vi "Phasor Measurement.vi"(0 "data in":T3, 1 "frequency configuration":T1={"channel index"=0, "nominal Fs/actual Fs"=1.0}, 2 "reset? (F)":bool, 7 "max time error [s]":dbl=1e-07 format="%#_15f", 9 "system info in":refnum<class "PMU System Info.lvclass">, 11 "error in (no error)":errorcluster, 12 "GPS information":T5[](array[typedef])) -> (3 "samples to read":u32, 4 "reporting data":T2 {"frequency" format="%#.6g"}, 6 "reporting timing information":T4 {"time quality flag" format="%.0b"}, 10 "system info out":refnum<class "PMU System Info.lvclass">, 14 "physical phasors":csg[](array[numeric]), 15 "error out":errorcluster)   [LabVIEW 2013, in "NI_EP_PMU.lvlib"]
doc: "LabVIEW no longer supports this VI. Use the Phasor Measurement (Std 2011) VI instead.\n\nCalculates the phasors, frequency, and frequency rate-of-change at the reporting timestamp according to IEEE Std C37.118-2005. This VI also returns the reported timestamp and other timing information for the fields in data frame, configuration frame, header frame, and command frame, as defined in IEEE Std C37.118-2005."
uses:
  <vilib>/addons/Electrical Power/PMU/NI_EP_PMU.lvlib
  <vilib>/addons/Electrical Power/PMU/Common/Classes/PMU System Info/PMU System Info.lvclass
  <vilib>/addons/Electrical Power/PMU/Common/Controls/pmu_GPS Info.ctl
  <vilib>/addons/Electrical Power/PMU/Common/Controls/pmu_Reporting Time Information.ctl
  <vilib>/addons/Electrical Power/PMU/Common/Controls/pmu_Phasor Measurement Data.ctl
  <vilib>/addons/Electrical Power/PMU/Common/Controls/pmu_Reporting Data.ctl
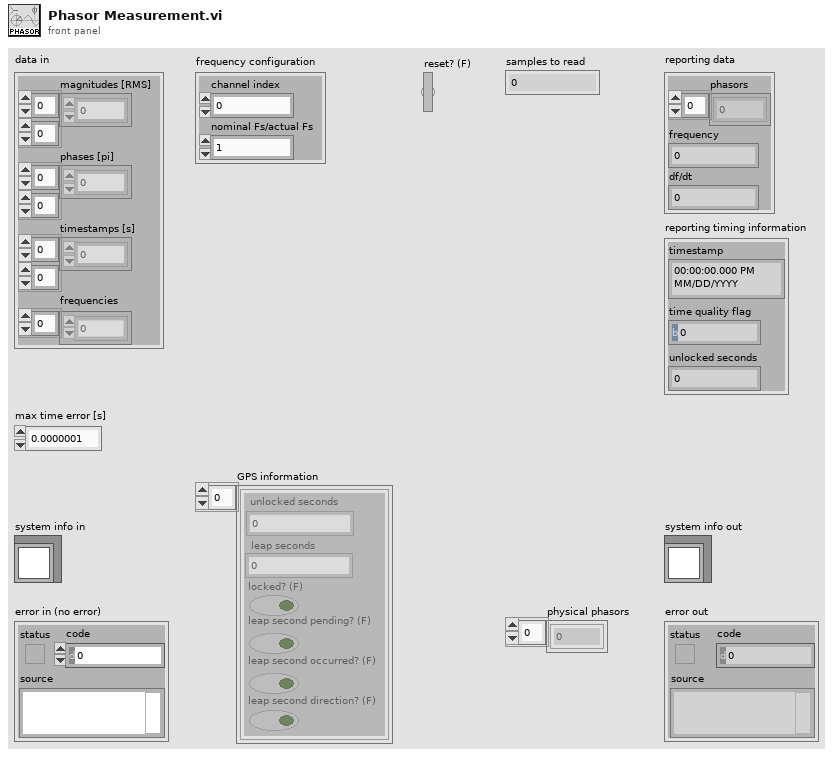
[diagram p1: front panel]
types:
  T1 = cluster{"channel index":i32, "nominal Fs/actual Fs":dbl}
  T2 = typedef "NI_EP_PMU.lvlib/pmu_Reporting Data.ctl" = cluster{"phasors":csg[], "frequency":sgl, "df/dt":sgl}
  T3 = typedef "NI_EP_PMU.lvlib/pmu_Phasor Measurement Data.ctl" = cluster{"magnitudes [RMS]":dbl[][], "phases [pi]":dbl[][], "timestamps [s]":dbl[][], "frequencies":dbl[]}
  T4 = typedef "NI_EP_PMU.lvlib/pmu_Reporting Time Information.ctl" = cluster{"time quality flag":u8, "unlocked seconds":u32, "timestamp":timestamp}
  T5 = typedef "NI_EP_PMU.lvlib/pmu_GPS Info.ctl" = cluster{"unlocked seconds":u32, "leap seconds":i8, "locked? (F)":bool, "leap second pending? (F)":bool, "leap second occurred? (F)":bool, "leap second direction? (F)":bool}
  T6 = cluster{"reporting timestamp":dbl[], "reporting magnitudes [RMS]":dbl[], "reporting phases [pi]":dbl[]}
  T7 = cluster{"zero-crossing timestamps [s]":dbl[], "zero-crossing frequencies":dbl[]}
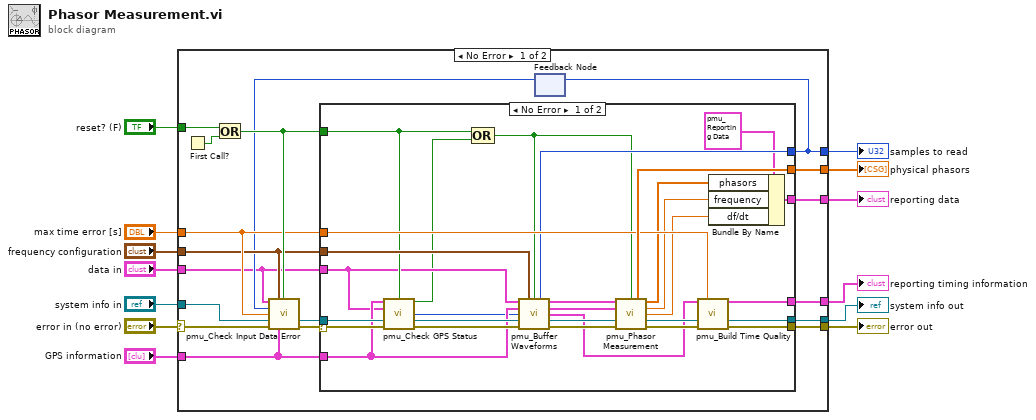
[diagram p0: block diagram]
diagram:
  n1 = case shown="No Error" "error in (no error)" {
    selector: "error in (no error)" -> [w18 w64]
    tunnel: "data in" -> [w14 _]
    tunnel: "system info in" -> [w23 w63]
    tunnel: [w31 _] -> w11
    tunnel: [w30 w63] -> w2
    tunnel: [w29 w64] -> w10
    tunnel: [w28 _] -> w9
    tunnel: "max time error [s]" -> [w24 _]
    tunnel: "frequency configuration" -> [w20 _]
    tunnel: [w16 _] -> w6
    tunnel: "GPS information" -> [w21 _]
    tunnel: "reset? (F)" -> [w26 _]
    tunnel: [w15 _] -> w1
    frame No Error {
      n2 = First Call?() -> (First Call?: T/F=w27:bool)
      n3 = Or(x=w26, y=w27) -> (x .or. y?=w25:bool)
      n4 = feedback #1() -> (w17:u32)  [unwired: 1 in]
      n5 = call <vilib>:"pmu_Check Input Data Error.vi"("data in"=w14, "frequency configuration"=w20, "reset? (F)"=w25, "elements need to read"=w17, "max time error [s]"=w24, "system info in"=w23, "error in (no error)"=w18, "GPS information"=w21) -> ("system info out"=w22:refnum<class "PMU System Info.lvclass">, "error out"=w19:errorcluster)  [unwired: 6 in]
      n6 = case shown="No Error" w19 {
        selector: w19 -> [w44 w62]
        tunnel: w14 -> [w33 _]
        tunnel: [w58 _] -> w31
        tunnel: [w57 w61] -> w30
        tunnel: [w56 w62] -> w29
        tunnel: [w55 _] -> w28
        tunnel: w24 -> [w52 _]
        tunnel: w20 -> [w50 _]
        tunnel: [w42 _] -> w16
        tunnel: w21 -> [w43 _]
        tunnel: w25 -> [w36 _]
        tunnel: w22 -> [w46 w61]
        tunnel: [w37 _] -> w15
        frame No Error {
          n7 = call <vilib>:"pmu_Check GPS Status.vi"("GPS information"=w43, "reset? (F)"=w36, "data in"=w33, "system info in"=w46, "error in (no error)"=w44) -> ("GPS first locking?"=w32:bool, "unlocked first index"=w34:i32, "system info out"=w47:refnum<class "PMU System Info.lvclass">, "error out"=w48:errorcluster)  [unwired: 7 in]
          n8 = Compound Arithmetic op=OR(w36, w32) -> (w35:bool)
          n9 = call <vilib>:"pmu_Buffer Waveforms.vi"("data in"=w33, "frequency configuration"=w50, "reset? (F)"=w35, "GPS information"=w43, "unlocked first index"=w34, "system info in"=w47, "error in (no error)"=w48) -> ("samples to read"=w42:u32, "reporting raw data"=w49:T6, "buffered zero-crossing frequency"=w51:T7, "reporting GPS information"=w45:T5, "system info out"=w60:refnum<class "PMU System Info.lvclass">, "error out"=w59:errorcluster)  [unwired: 3 in]
          n10 = call <vilib>:"pmu_Phasor Measurement.vi"("reporting raw data"=w49, "reset? (F)"=w35, "buffered zero-crossing frequencies"=w51, "system info in"=w60, "error in (no error)"=w59) -> ("physical phasors"=w58:csg[], "reporting phasors"=w40:csg[], "reporting frequency"=w39:sgl, "reporting df/dt"=w38:sgl, "system info out"=w54:refnum<class "PMU System Info.lvclass">, "error out"=w53:errorcluster)  [unwired: 5 in]
          n11 = call <vilib>:"pmu_Build Time Quality.vi"("reported GPS information"=w45, "max time error [s]"=w52, "system info in"=w54, "error in (no error)"=w53) -> ("reporting timing information"=w55:T4, "system info out"=w57:refnum<class "PMU System Info.lvclass">, "error out"=w56:errorcluster)  [unwired: 9 in]
          n12 = Bundle By Name(cluster=T2 {"phasors"=[0.011429072-99.96636i, -86.60898+49.966427i, 86.59466+50.004635i, 0.00039273032-0.9994094i, 0.00039950816-0.9995112i, 0.00037330666-0.9995143i], "frequency"=49.999996, "df/dt"=0.00031614315} ("reporting data"), "phasors"=w40, "frequency"=w39, "df/dt"=w38) -> (w37:T2)
        }
        frame Error {
        }
      }
      n13 = feedback-in #1(w16) -> ()
    }
    frame Error {
    }
  }
  "error out" <- w10
  "system info out" <- w2
  "reporting timing information" <- w9
  "reporting data" <- w1
  "physical phasors" <- w11
  "samples to read" <- w6
